vi "Load Board Power.vi"(0 "TSM context":T1, 5 "+5 V power enabled":bool, 7 "+15 V power enabled":bool, 9 "-15 V power enabled":bool, 11 "+30 V power enabled":bool, 12 "+12 V power enabled":bool, 13 "+48 V power enabled":bool) -> (15 "error out":errorcluster)   [LabVIEW 2020]
uses:
  <vilib>/NI_TestStand_SemiconductorModule/NI_TestStand_Semiconductor_Module.lvlibp/PinMap/General/SemiconductorModuleContext.ctl
  dd3c7301-949c-4674-90e5-aa35a0d37f3c.vi
  dd3c7301-949c-4674-90e5-aa35a0d37f3c.vi/5b476390-81d5-47ce-b096-475617707f02.vi
  dd3c7301-949c-4674-90e5-aa35a0d37f3c.vi/e4ff030e-b680-461e-8ce6-d49452e77caf.vi
  dd3c7301-949c-4674-90e5-aa35a0d37f3c.vi/dfd6eb5f-8e6d-417f-b74b-acbbb2f7fb34.vi
  dd3c7301-949c-4674-90e5-aa35a0d37f3c.vi/b2c73eed-24f6-4569-8f62-5ef2dac11b10.vi
  dd3c7301-949c-4674-90e5-aa35a0d37f3c.vi/dfd6eb5f-8e6d-417f-b74b-acbbb2f7fb34.vi/9bc7fa08-00ae-4276-8790-10e6602cd148.vi
  Instrument Control/Shared SubVIs/Trim Whitespace [Inlined].vi
  Instrument Control/DCPower/SubVIs/SSC DCPower Expanded Pin List to SSC Index.vi
  Instrument Control/Shared SubVIs/Channel List to Pins.vi
  <vilib>/Utility/error.llb/Error Cluster From Error Code.vi
  Instrument Control/DCPower/SSC DCPower/Source/Constant Voltage/SSC DCPower Force Voltage Array Symmetric Limits.vi
  <vilib>/NI_STS_Maintenance_API/NI_STS_Maintenance_API.lvlibp/subVIs/Write Settings/niSTS Write Enable 48V Power.vi
  <vilib>/NI_STS_Maintenance_API/NI_STS_Maintenance_API.lvlibp/subVIs/Write Settings/niSTS Write Enable 12V DIB Power.vi
  <vilib>/NI_STS_Maintenance_API/NI_STS_Maintenance_API.lvlibp/niSTS Monitoring API.lvclass
  <vilib>/NI_STS_Maintenance_API/NI_STS_Maintenance_API.lvlibp
  <vilib>/NI_TestStand_SemiconductorModule/NI_TestStand_Semiconductor_Module.lvlibp
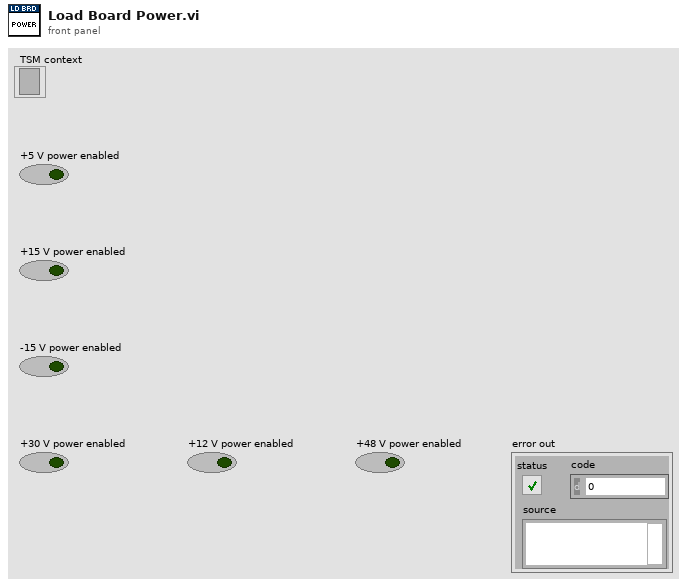
[diagram p1: front panel]
types:
  T1 = typedef "NI_TestStand_Semiconductor_Module.lvlibp/SemiconductorModuleContext.ctl" = refnum<k7>
  T2 = typedef "TSM SSC DCPower.ctl" = cluster{"Pin Query Context":refnum<class "MultiplePinMultipleSessionQueryContext.lvclass">, "SSC":T3[], "Site Numbers":i32[], "Pins":T4[], "Pins Expanded":T6[]}
  T3 = typedef "SSC DCPower.ctl" = cluster{"Session":refnum<k15>, "Chan":string, "Channel List":string}
  T4 = typedef "TSM Pin Information.ctl" = cluster{"Pin":tag, "Type":T5, "Count":i32}
  T5 = typedef "TSM Pin Type Identifier.ctl" = enum8{"DUT Pin", "System Pin", "Pin Group", "Not Determined"}
  T6 = typedef "TSM Expanded Pin Information.ctl" = cluster{"Pin":tag, "Type":T5, "Index":i32}
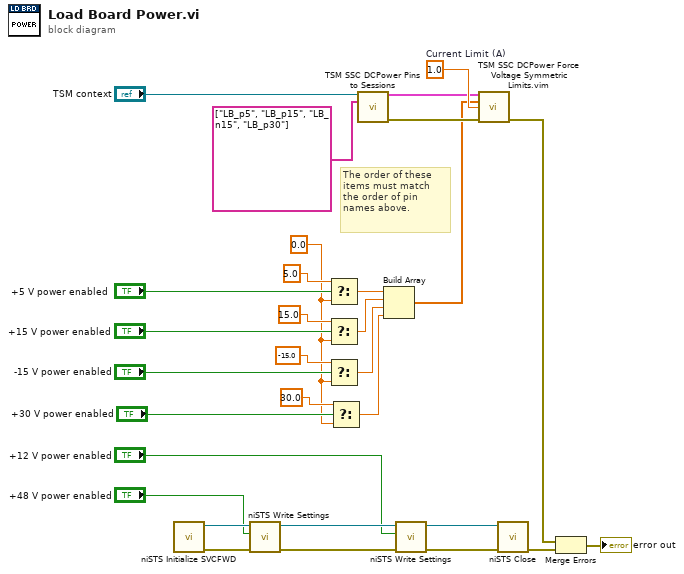
[diagram p0: block diagram]
diagram:
  w2 = 0.0 ("f")
  w27 = 1.0  # Current Limit (A)
  # "The order of these items must match the order of pin names above."
  n1 = call <vilib>:"niSTS Initialize SVCFWD.vi"() -> ("error out"=w17:errorcluster, "STS Maintence API Session (out)"=w18:refnum<class "niSTS Monitoring API.lvclass">)  [unwired: 10 in]
  n2 = call-poly <vilib>:"niSTS Write Settings.vi"("error in"=w17, "Enable DIB 48V"="+48 V power enabled", "STS Maintence API Session (in)"=w18) -> ("error out"=w14:errorcluster, "STS Maintence API Session (out)"=w15:refnum<class "niSTS Monitoring API.lvclass">)  [unwired: 6 in, 1 out]
  n3 = Select(t=5.0, s="+5 V power enabled", f=w2) -> (s? t:f=w25:dbl)
  n4 = Select(t=15.0, s="+15 V power enabled", f=w2) -> (s? t:f=w8:dbl)
  n5 = Select(t=-15.0, s="-15 V power enabled", f=w2) -> (s? t:f=w7:dbl)
  n6 = Select(t=30.0, s="+30 V power enabled", f=w2) -> (s? t:f=w1:dbl)
  n7 = call "TSM SSC DCPower Pins to Sessions.vi"("TSM context"="TSM context", "Pins"=tag[] ["LB_p5", "LB_p15", "LB_n15", "LB_p30"]) -> ("DCPower TSM Out"=w5:T2, "error out"=w28:errorcluster)  [unwired: 12 in]
  n8 = Build Array(w25, w8, w7, w1) -> (w9:dbl[])
  n9 = call-poly <vilib>:"niSTS Write Settings.vi"("error in"=w14, "Enable DIB 12V"="+12 V power enabled", "STS Maintence API Session (in)"=w15) -> ("error out"=w13:errorcluster, "STS Maintence API Session (out)"=w12:refnum<class "niSTS Monitoring API.lvclass">)  [unwired: 6 in, 1 out]
  n10 = call "TSM SSC DCPower Force Voltage Symmetric Limits.vim"("DCPower TSM in"=w5, "Voltage Level (V)"=w9, "Current Limit (A)"=w27, "error in"=w28) -> ("error out"=w19:errorcluster)  [unwired: 10 in, 1 out]
  n11 = call <vilib>:"niSTS Close.vi"("error in"=w13, "STS Maintence API Session (in)"=w12) -> ("error out"=w11:errorcluster)  [unwired: 9 in]
  n12 = Merge Errors(w19, w11) -> (→"error out":errorcluster)
